vi "Keithley6487_setrange.vi"(8 "error in (no error)":errorcluster, 9 "Enum":T1(ring), 11 "VISA resource name":refnum<visa-resource-name>) -> (0 "error out":errorcluster, 3 "VISA resource name out":refnum<visa-resource-name>)   [LabVIEW 2016]
panel:
  out "resulting string":string
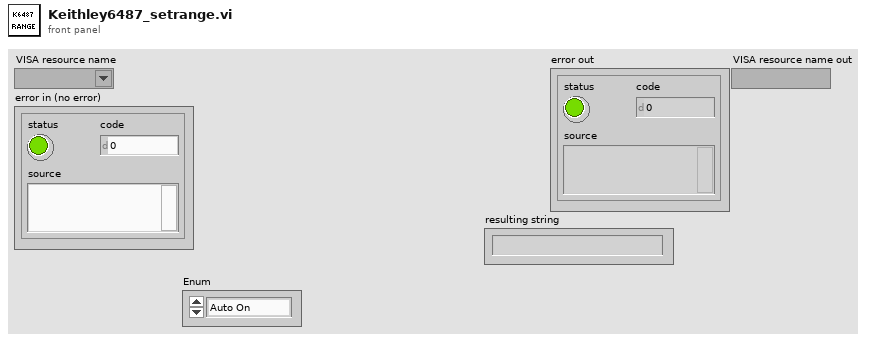
[diagram p1: front panel]
types:
  T1 = enum16{"Auto On", "2e-9", "2e-8", "2e-7", "2e-6", "2e-5", "2e-4", "2e-3", "2e-2"}
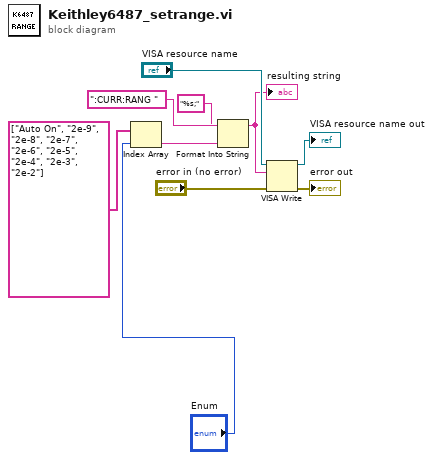
[diagram p0: block diagram]
diagram:
  n1 = Index Array(array=string[] ["Auto On", "2e-9", "2e-8", "2e-7", "2e-6", "2e-5", "2e-4", "2e-3", "2e-2"], index="Enum") -> (element=w4:string)
  n2 = Format Into String(format string="%s;" ("write buffer"), initial string=":CURR:RANG " ("write buffer"), w4) -> (resulting string=w2:string)  [unwired: 1 in, 1 out]
  "resulting string" <- w2
  n3 = VISA Write(VISA resource name="VISA resource name", write buffer=w2, error in (no error)="error in (no error)") -> (VISA resource name out=→"VISA resource name out":refnum<visa-resource-name>, error out=→"error out":errorcluster)  [unwired: 1 out]
